vi "Stop Process.vi"(0 "Process In":refnum<class "Process.lvclass">, 7 "Timeout in ms (-1)":i32=-1, 11 "Error In":errorcluster) -> (4 "Process Out":refnum<class "Process.lvclass">, 15 "Error Out":errorcluster)   [LabVIEW 2023, in "Process.lvclass"]
doc: "Sends Close command to process, waits Timeout for confirmation then destroys queues associated with process. If process is unresponsive, aborts it."
uses:
  Process.lvclass
  Interfaces/ICanCommunicate/Message.ctl
  Interfaces/ICanCommunicate/ICanCommunicate.lvclass
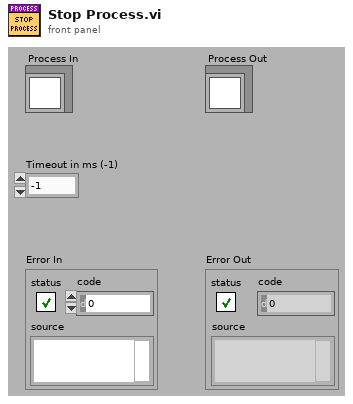
[diagram p1: front panel]
types:
  T1 = enum16{"ReadRepository", "CreateNew", "CreateOrLookUpExisting", "ReadRepositoryAndDestroy"}
  T2 = typedef "ICanCommunicate.lvclass/ToProcessQueue.ctl" = refnum<queue>
  T3 = typedef "ICanCommunicate.lvclass/ProcessSyncQueue.ctl" = refnum<queue>
  T4 = typedef "ICanCommunicate.lvclass/FromProcessQueue.ctl" = refnum<queue>
  T5 = typedef "ICanCommunicate.lvclass/Message.ctl" = cluster{"Sender Name":string, "Recipent Name":string, "Command":string, "Data":variant, "Time Stamp":timestamp, "GUID":string, "Chcecksum":string}
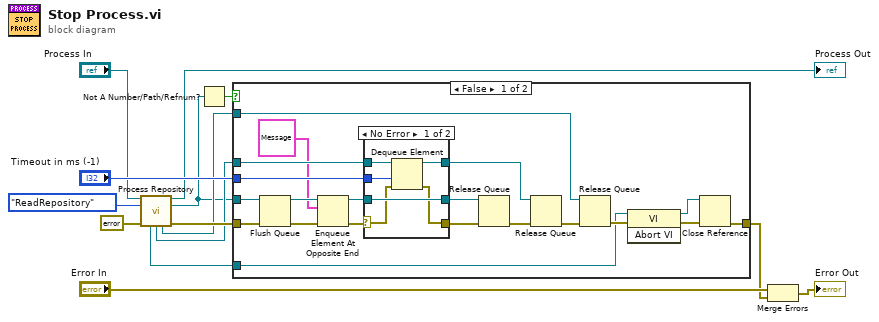
[diagram p0: block diagram]
diagram:
  n1 = call-dynamic "Process Repository.vi"("Process In"="Process In", "Action(ReadRepository)"=T1."ReadRepository", "Error In"=errorcluster {"status"=FALSE, "code"=0, "source"=""} ("error in (no error)")) -> ("Process Out"=→"Process Out":refnum<class "Process.lvclass">, "ToProcessQueue"=w3:T2, "ProcessViRef"=w5:refnum<vi>, "ProcessSyncQueue"=w7:T3, "FromProcessQueue"=w6:T4, "Error Out"=w8:errorcluster)  [unwired: 6 in, 1 out]
  n2 = Not A Number/Path/Refnum?(number/path/refnum=w3) -> (NaN/Path/Refnum?=w2:bool)
  n3 = case shown="False" w2 {
    tunnel: w7 -> [w30 _]
    tunnel: w8 -> [w31 w44]
    tunnel: [w26 w44] -> w12
    tunnel: w3 -> [w34 _]
    tunnel: "Timeout in ms (-1)" -> [w25 _]
    tunnel: w6 -> [w23 _]
    tunnel: w5 -> [w17 _]
    frame False {
      n4 = Flush Queue(queue=w34, error in (no error)=w31) -> (queue out=w32:T2, error out=w33:errorcluster)  [unwired: 1 out]
      n5 = Enqueue Element At Opposite End(queue=w32, element=T5 {"Sender Name"="", "Recipent Name"="", "Command"="Close", "Data"=variant, "Time Stamp"=timestamp(0 s since 1904-01-01), "GUID"="", "Chcecksum"=""} ("Message"), error in (no error)=w33) -> (queue out=w29:T2, error out=w24:errorcluster)  [unwired: 1 in, 1 out]
      n6 = case shown="No Error" w24 {
        tunnel: [w36 w43] -> w28
        tunnel: w30 -> [w39 w41]
        tunnel: [w40 w42] -> w27
        tunnel: w29 -> [w40 w42]
        tunnel: w25 -> [w38 _]
        selector: w24 -> [w37 w43]
        tunnel: [w35 w41] -> w21
        frame No Error {
          n7 = Dequeue Element(queue=w39, timeout in ms (-1)=w38, error in (no error)=w37) -> (queue out=w35:T3, error out=w36:errorcluster)  [unwired: 2 out]
        }
        frame Error {
        }
      }
      n8 = Release Queue(queue=w27, error in (no error)=w28) -> (error out=w22:errorcluster)  [unwired: 1 in, 2 out]
      n9 = Release Queue(queue=w21, error in (no error)=w22) -> (error out=w20:errorcluster)  [unwired: 1 in, 2 out]
      n10 = Release Queue(queue=w23, error in (no error)=w20) -> (error out=w19:errorcluster)  [unwired: 1 in, 2 out]
      n11 = invoke class="VI" method="Abort VI"(reference=w17, error in=w19) -> (reference out=w16:refnum<vi>, error out=w18:errorcluster)  [unwired: 1 in, 1 out]
      n12 = Close Reference(reference=w16, error in (no error)=w18) -> (error out=w26:errorcluster)
    }
    frame True {
    }
  }
  n13 = Merge Errors("Error In", w12) -> (→"Error Out":errorcluster)
